vi "OE_Mis_time.vi"(7 "Seelected date":timestamp=timestamp(3772872308.6086583 s since 1904-01-01), 8 "error in (no error)":errorcluster, 10 "Cluster in":T1={"connection reference"=refnum, "Net Avai time (Min)"=0, "pLAN dATE datA"=[], "Data by plan date, shift, product"=[], "BreakDownd Data"=[], "Raw rejection Data"=[], "mislanius times shift 1"={"Lunch Time From"=timestamp(3772871904.6410136 s since 1904-01-01), "Lunch Time To"=timestamp(3772871909.6739416 s since 1904-01-01), "Tea Time From"=timestamp(3772871914.1118393 s since 1904-01-01), "Tea Time To"=timestamp(3772871912.0217314 s since 1904-01-01), "Clean Time From"=timestamp(3772871918.5572615 s since 1904-01-01), "Clean Time To"=timestamp(3772871916.1777034 s since 1904-01-01), "Meeting Time From"=timestamp(3772871920.7462983 s since 1904-01-01), "Meeting Time To"=timestamp(3772871922.664581 s since 1904-01-01), "Dev/Other Time From"=timestamp(3772871924.9359455 s since 1904-01-01), "Dev/Other Time To"=timestamp(3772871926.9172926 s since 1904-01-01), "Meeting"=TRUE, "Dev/Other"=TRUE}, "mislanius times shift 2"={"Lunch Time From"=timestamp(3772871937.417959 s since 1904-01-01), "Lunch Time To"=timestamp(3772871939.5655127 s since 1904-01-01), "Tea Time From"=timestamp(3772871941.53232 s since 1904-01-01), "Tea Time To"=timestamp(3772871944.2390895 s since 1904-01-01), "Clean Time From"=timestamp(3772871947.9368706 s since 1904-01-01), "Clean Time To"=timestamp(3772871950.09432 s since 1904-01-01), "Meeting Time From"=timestamp(3772871952.5211887 s since 1904-01-01), "Meeting Time To"=timestamp(3772871954.4985256 s since 1904-01-01), "Dev/Other Time From"=timestamp(3772871934.6783137 s since 1904-01-01), "Dev/Other Time To"=timestamp(3772871932.403295 s since 1904-01-01), "Meeting"=TRUE, "Dev/Other"=TRUE}} {"mislanius times shift 2"."Lunch Time From" format="%<%.X %x>T"; "mislanius times shift 2"."Lunch Time To" format="%<%.X %x>T"; "mislanius times shift 2"."Tea Time From" format="%<%.X %x>T"; "mislanius times shift 2"."Tea Time To" format="%<%.X %x>T"; "mislanius times shift 2"."Clean Time From" format="%<%.X %x>T"; "mislanius times shift 2"."Clean Time To" format="%<%.X %x>T"; "mislanius times shift 2"."Meeting Time From" format="%<%.X %x>T"; "mislanius times shift 2"."Meeting Time To" format="%<%.X %x>T"; "mislanius times shift 2"."Dev/Other Time From" format="%<%.X %x>T"; "mislanius times shift 2"."Dev/Other Time To" format="%<%.X %x>T"; "mislanius times shift 1"."Lunch Time From" format="%<%.X %x>T"; "mislanius times shift 1"."Lunch Time To" format="%<%.X %x>T"; "mislanius times shift 1"."Tea Time From" format="%<%.X %x>T"; "mislanius times shift 1"."Tea Time To" format="%<%.X %x>T"; "mislanius times shift 1"."Clean Time From" format="%<%.X %x>T"; "mislanius times shift 1"."Clean Time To" format="%<%.X %x>T"; "mislanius times shift 1"."Meeting Time From" format="%<%.X %x>T"; "mislanius times shift 1"."Meeting Time To" format="%<%.X %x>T"; "mislanius times shift 1"."Dev/Other Time From" format="%<%.X %x>T"; "mislanius times shift 1"."Dev/Other Time To" format="%<%.X %x>T"}, 11 "appended path":path) -> (0 "error out":errorcluster, 1 "Cluster out":T1={"connection reference"=refnum, "Net Avai time (Min)"=0, "pLAN dATE datA"=[], "Data by plan date, shift, product"=[], "BreakDownd Data"=[], "Raw rejection Data"=[], "mislanius times shift 1"={"Lunch Time From"=timestamp(0 s since 1904-01-01), "Lunch Time To"=timestamp(0 s since 1904-01-01), "Tea Time From"=timestamp(0 s since 1904-01-01), "Tea Time To"=timestamp(0 s since 1904-01-01), "Clean Time From"=timestamp(0 s since 1904-01-01), "Clean Time To"=timestamp(0 s since 1904-01-01), "Meeting Time From"=timestamp(0 s since 1904-01-01), "Meeting Time To"=timestamp(0 s since 1904-01-01), "Dev/Other Time From"=timestamp(0 s since 1904-01-01), "Dev/Other Time To"=timestamp(0 s since 1904-01-01), "Meeting"=FALSE, "Dev/Other"=TRUE}, "mislanius times shift 2"={"Lunch Time From"=timestamp(0 s since 1904-01-01), "Lunch Time To"=timestamp(0 s since 1904-01-01), "Tea Time From"=timestamp(0 s since 1904-01-01), "Tea Time To"=timestamp(0 s since 1904-01-01), "Clean Time From"=timestamp(0 s since 1904-01-01), "Clean Time To"=timestamp(0 s since 1904-01-01), "Meeting Time From"=timestamp(0 s since 1904-01-01), "Meeting Time To"=timestamp(0 s since 1904-01-01), "Dev/Other Time From"=timestamp(0 s since 1904-01-01), "Dev/Other Time To"=timestamp(0 s since 1904-01-01), "Meeting"=FALSE, "Dev/Other"=TRUE}} {"mislanius times shift 2"."Lunch Time From" format="%<%.X %x>T"; "mislanius times shift 2"."Lunch Time To" format="%<%.X %x>T"; "mislanius times shift 2"."Tea Time From" format="%<%.X %x>T"; "mislanius times shift 2"."Tea Time To" format="%<%.X %x>T"; "mislanius times shift 2"."Clean Time From" format="%<%.X %x>T"; "mislanius times shift 2"."Clean Time To" format="%<%.X %x>T"; "mislanius times shift 2"."Meeting Time From" format="%<%.X %x>T"; "mislanius times shift 2"."Meeting Time To" format="%<%.X %x>T"; "mislanius times shift 2"."Dev/Other Time From" format="%<%.X %x>T"; "mislanius times shift 2"."Dev/Other Time To" format="%<%.X %x>T"; "mislanius times shift 1"."Lunch Time From" format="%<%.X %x>T"; "mislanius times shift 1"."Lunch Time To" format="%<%.X %x>T"; "mislanius times shift 1"."Tea Time From" format="%<%.X %x>T"; "mislanius times shift 1"."Tea Time To" format="%<%.X %x>T"; "mislanius times shift 1"."Clean Time From" format="%<%.X %x>T"; "mislanius times shift 1"."Clean Time To" format="%<%.X %x>T"; "mislanius times shift 1"."Meeting Time From" format="%<%.X %x>T"; "mislanius times shift 1"."Meeting Time To" format="%<%.X %x>T"; "mislanius times shift 1"."Dev/Other Time From" format="%<%.X %x>T"; "mislanius times shift 1"."Dev/Other Time To" format="%<%.X %x>T"})   [LabVIEW 2017]
uses:
  Controls/OE_screen_cluster.ctl
  <vilib>/addons/database/Connection.llb/Conn ObjectReference.ctl
  <vilib>/addons/database/NI_Database_API.lvlib
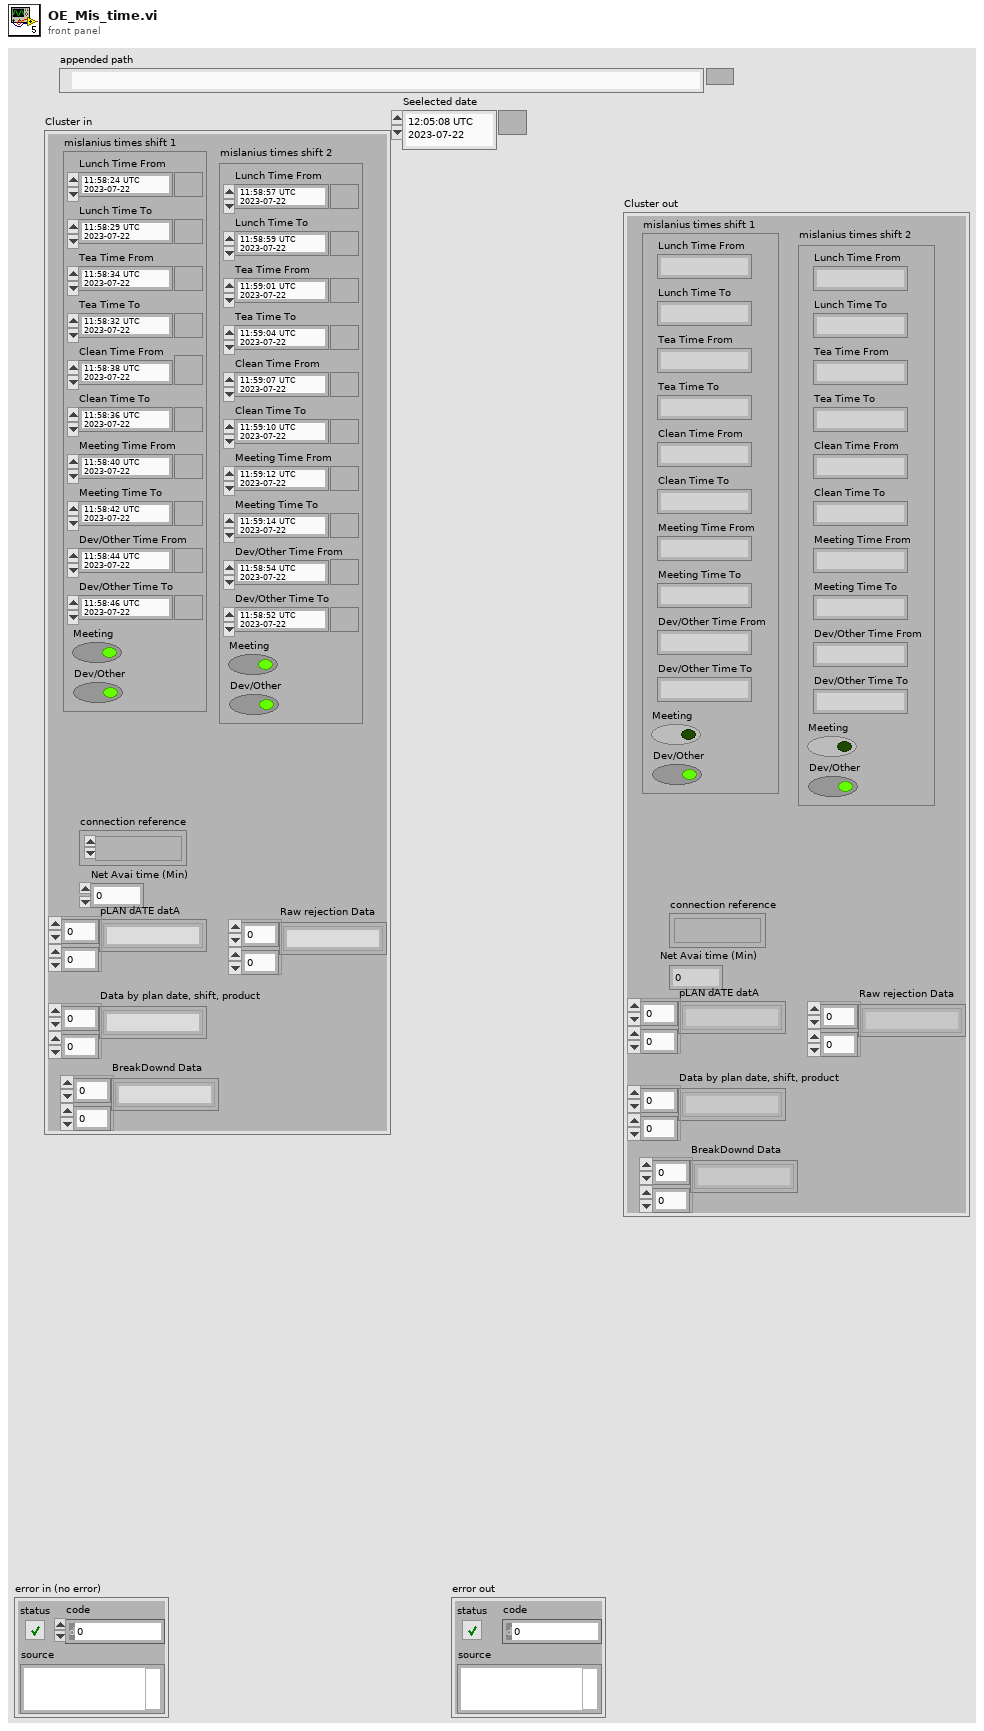
[diagram p1: front panel]
types:
  T1 = typedef "OE_screen_cluster.ctl" = cluster{"connection reference":T2, "Net Avai time (Min)":i32, "pLAN dATE datA":string[][], "Data by plan date, shift, product":string[][], "BreakDownd Data":string[][], "Raw rejection Data":string[][], "mislanius times shift 1":cluster{"Lunch Time From":timestamp, "Lunch Time To":timestamp, "Tea Time From":timestamp, "Tea Time To":timestamp, "Clean Time From":timestamp, "Clean Time To":timestamp, "Meeting Time From":timestamp, "Meeting Time To":timestamp, "Dev/Other Time From":timestamp, "Dev/Other Time To":timestamp, "Meeting":bool, "Dev/Other":bool}, "mislanius times shift 2":cluster{"Lunch Time From":timestamp, "Lunch Time To":timestamp, "Tea Time From":timestamp, "Tea Time To":timestamp, "Clean Time From":timestamp, "Clean Time To":timestamp, "Meeting Time From":timestamp, "Meeting Time To":timestamp, "Dev/Other Time From":timestamp, "Dev/Other Time To":timestamp, "Meeting":bool, "Dev/Other":bool}}
  T2 = typedef "NI_Database_API.lvlib/Conn ObjectReference.ctl" = refnum<k1>
  T3 = enum16{"open", "replace", "create", "open or create", "replace or create", "replace or create with confirmation"}
  T4 = cluster{"unsigned 64bit integer":u64, "unsigned 64bit integer 2":u64, "unsigned 64bit integer 3":u64, "unsigned 64bit integer 4":u64, "unsigned 64bit integer 5":u64, "unsigned 64bit integer 6":u64, "unsigned 64bit integer 7":u64, "unsigned 64bit integer 8":u64, "unsigned 64bit integer 9":u64, "unsigned 64bit integer 10":u64, "Meeting":bool, "Dev/other 1":bool, "unsigned 64bit integer 11":u64, "unsigned 64bit integer 12":u64, "unsigned 64bit integer 13":u64, "unsigned 64bit integer 14":u64, "unsigned 64bit integer 15":u64, "unsigned 64bit integer 16":u64, "unsigned 64bit integer 17":u64, "unsigned 64bit integer 18":u64, "unsigned 64bit integer 19":u64, "unsigned 64bit integer 20":u64, "Meeting 2":bool, "Dev/other 2":bool}
  T5 = cluster{"Lunch Time From":timestamp, "Lunch Time To":timestamp, "Tea Time From":timestamp, "Tea Time To":timestamp, "Clean Time From":timestamp, "Clean Time To":timestamp, "Meeting Time From":timestamp, "Meeting Time To":timestamp, "Dev/Other Time From":timestamp, "Dev/Other Time To":timestamp, "Meeting":bool, "Dev/Other":bool}
  T6 = typedef "LVDateTimeRec.ctl" = cluster{"fractional second":dbl, "second":i32, "minute":i32, "hour":i32, "day of month":i32, "month":i32, "year":i32, "day of week":i32, "day of year":i32, "DST":i32}
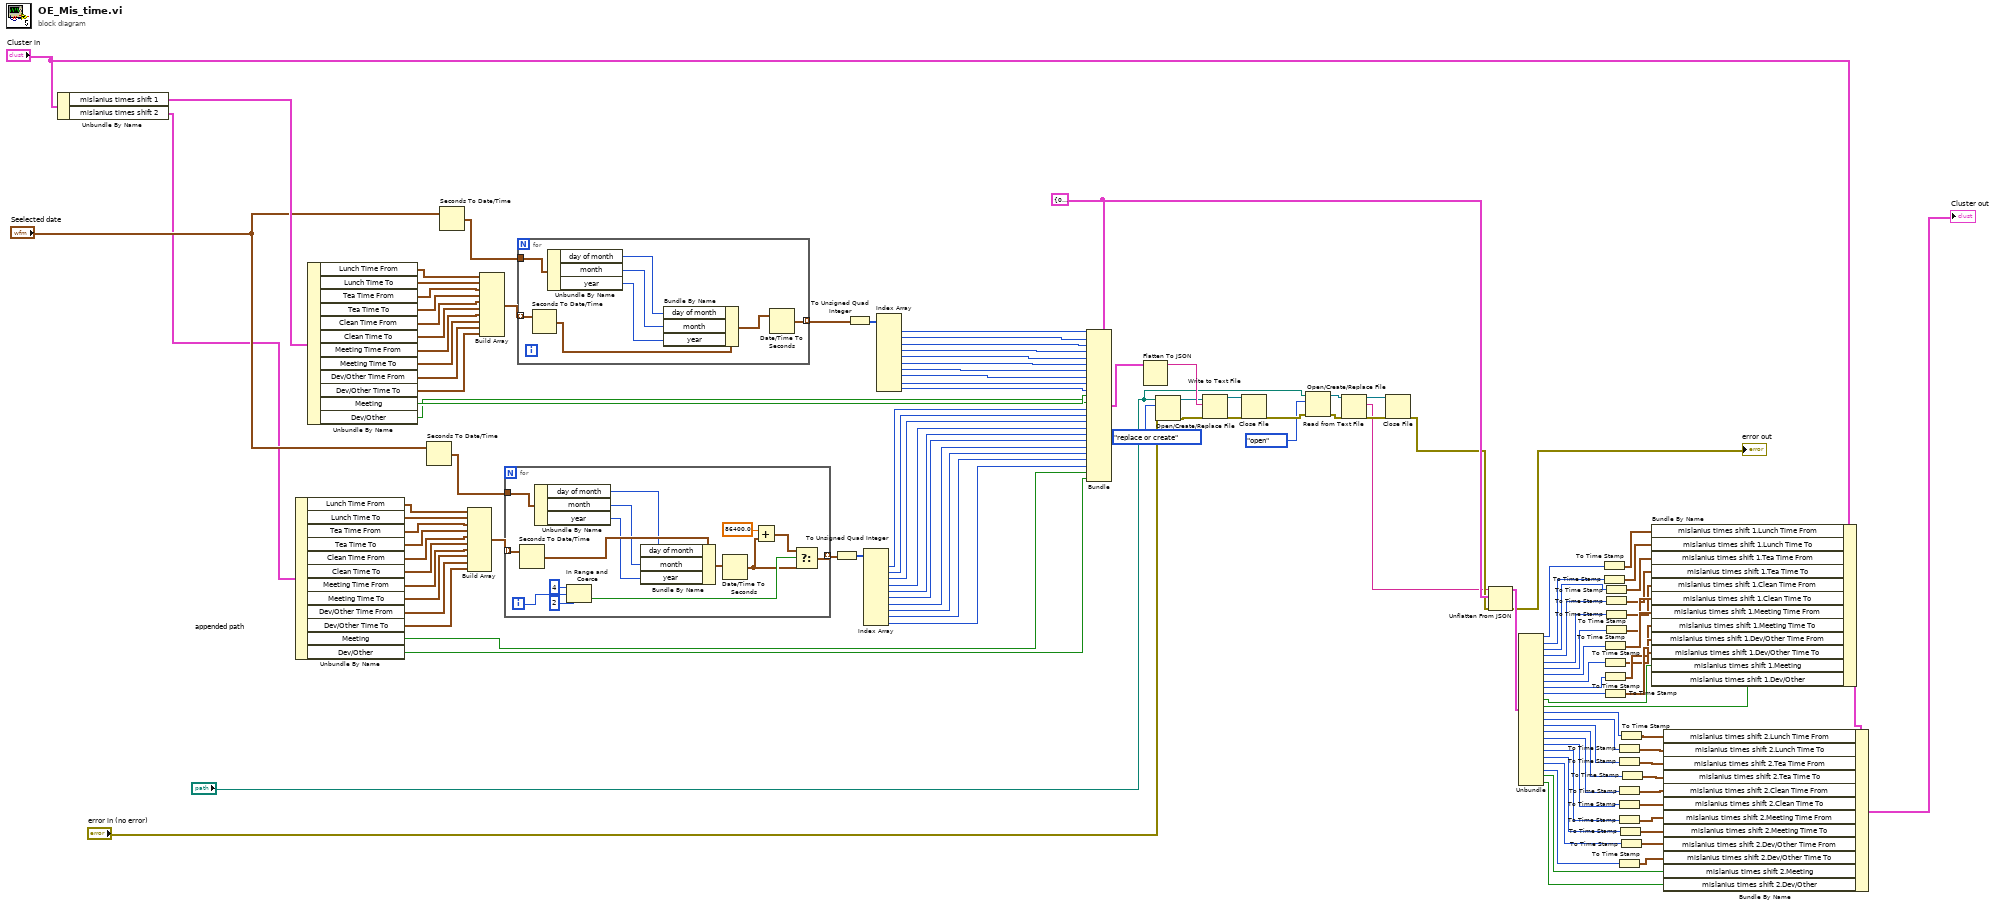
[diagram p0: block diagram]
diagram:
  w93 = T4 {"unsigned 64bit integer"=0, "unsigned 64bit integer 2"=0, "unsigned 64bit integer 3"=0, "unsigned 64bit integer 4"=0, "unsigned 64bit integer 5"=0, "unsigned 64bit integer 6"=0, "unsigned 64bit integer 7"=0, "unsigned 64bit integer 8"=0, "unsigned 64bit integer 9"=0, "unsigned 64bit integer 10"=0, "Meeting"=FALSE, "Dev/other 1"=FALSE, "unsigned 64bit integer 11"=0, "unsigned 64bit integer 12"=0, "unsigned 64bit integer 13"=0, "unsigned 64bit integer 14"=0, "unsigned 64bit integer 15"=0, "unsigned 64bit integer 16"=0, "unsigned 64bit integer 17"=0, "unsigned 64bit integer 18"=0, "unsigned 64bit integer 19"=0, "unsigned 64bit integer 20"=0, "Meeting 2"=FALSE, "Dev/other 2"=FALSE} ("input cluster")
  n1 = Unbundle By Name("Cluster in") -> ("mislanius times shift 1"=w81:T5, "mislanius times shift 2"=w41:T5)
  n2 = Unbundle By Name(w41) -> ("Lunch Time From"=w43:timestamp, "Lunch Time To"=w45:timestamp, "Tea Time From"=w46:timestamp, "Tea Time To"=w47:timestamp, "Clean Time From"=w48:timestamp, "Clean Time To"=w49:timestamp, "Meeting Time From"=w50:timestamp, "Meeting Time To"=w51:timestamp, "Dev/Other Time From"=w52:timestamp, "Dev/Other Time To"=w53:timestamp, "Meeting"=w38:bool, "Dev/Other"=w37:bool)
  n3 = Unbundle By Name(w81) -> ("Lunch Time From"=w80:timestamp, "Lunch Time To"=w78:timestamp, "Tea Time From"=w77:timestamp, "Tea Time To"=w76:timestamp, "Clean Time From"=w75:timestamp, "Clean Time To"=w74:timestamp, "Meeting Time From"=w73:timestamp, "Meeting Time To"=w72:timestamp, "Dev/Other Time From"=w71:timestamp, "Dev/Other Time To"=w70:timestamp, "Meeting"=w40:bool, "Dev/Other"=w39:bool)
  n4 = Seconds To Date/Time(time stamp (now)="Seelected date") -> (date time rec=w54:T6)  [unwired: 1 in]
  n5 = Seconds To Date/Time(time stamp (now)="Seelected date") -> (date time rec=w69:T6)  [unwired: 1 in]
  n6 = Build Array(w43, w45, w46, w47, w48, w49, w50, w51, w52, w53) -> (w44:timestamp[])
  n7 = Build Array(w80, w78, w77, w76, w75, w74, w73, w72, w71, w70) -> (w79:timestamp[])
  n8 = for {
    tunnel: w44 -> [w135] mode=indexing
    tunnel: w54 -> [w127]
    tunnel: [w124] -> w55 mode=indexing
    i -> [w130]
    n9 = Seconds To Date/Time(time stamp (now)=w135) -> (date time rec=w137:T6)  [unwired: 1 in]
    n10 = Unbundle By Name(w127) -> ("day of month"=w129:i32, "month"=w134:i32, "year"=w133:i32)
    n11 = In Range and Coerce(upper limit=4, x=w130, lower limit=2) -> (In Range?=w126:bool)  [unwired: 1 out]
    n12 = Bundle By Name(cluster=w137, "day of month"=w129, "month"=w134, "year"=w133) -> (w136:T6)
    n13 = Date/Time To Seconds(2:w136) -> (0:w123:timestamp)  [unwired: 1 in]
    n14 = Add(x=86400.0 ("x-y 2"), y=w123) -> (x+y=w125:timestamp)
    n15 = Select(t=w125, s=w126, f=w123) -> (s? t:f=w124:timestamp)
  }
  n16 = for {
    tunnel: w79 -> [w143] mode=indexing
    tunnel: w69 -> [w142]
    tunnel: [w138] -> w68 mode=indexing
    n17 = Seconds To Date/Time(time stamp (now)=w143) -> (date time rec=w145:T6)  [unwired: 1 in]
    n18 = Unbundle By Name(w142) -> ("day of month"=w141:i32, "month"=w140:i32, "year"=w139:i32)
    n19 = Bundle By Name(cluster=w145, "day of month"=w141, "month"=w140, "year"=w139) -> (w144:T6)
    n20 = Date/Time To Seconds(2:w144) -> (0:w138:timestamp)  [unwired: 1 in]
  }
  n21 = To Unsigned Quad Integer(1:w55) -> (0:w56:u64[])
  n22 = To Unsigned Quad Integer(1:w68) -> (0:w67:u64[])
  n23 = Index Array(array=w56) -> (element #1=w27:u64, element #2=w28:u64, element #3=w29:u64, element #4=w30:u64, element #5=w31:u64, element #6=w32:u64, element #7=w33:u64, element #8=w34:u64, element #9=w35:u64, element #10=w36:u64)  [unwired: 10 in]
  n24 = Index Array(array=w67) -> (element #1=w66:u64, element #2=w65:u64, element #3=w64:u64, element #4=w63:u64, element #5=w62:u64, element #6=w61:u64, element #7=w60:u64, element #8=w59:u64, element #9=w58:u64, element #10=w57:u64)  [unwired: 10 in]
  n25 = Bundle(cluster=w93, "unsigned 64bit integer"=w66, "unsigned 64bit integer 2"=w65, "unsigned 64bit integer 3"=w64, "unsigned 64bit integer 4"=w63, "unsigned 64bit integer 5"=w62, "unsigned 64bit integer 6"=w61, "unsigned 64bit integer 7"=w60, "unsigned 64bit integer 8"=w59, "unsigned 64bit integer 9"=w58, "unsigned 64bit integer 10"=w57, "Meeting"=w40, "Dev/other 1"=w39, "unsigned 64bit integer 11"=w27, "unsigned 64bit integer 12"=w28, "unsigned 64bit integer 13"=w29, "unsigned 64bit integer 14"=w30, "unsigned 64bit integer 15"=w31, "unsigned 64bit integer 16"=w32, "unsigned 64bit integer 17"=w33, "unsigned 64bit integer 18"=w34, "unsigned 64bit integer 19"=w35, "unsigned 64bit integer 20"=w36, "Meeting 2"=w38, "Dev/other 2"=w37) -> (w118:T4)
  n26 = Flatten To JSON(anything=w118) -> (JSON string=w92:string)  [unwired: 2 in, 1 out]
  n27 = Open/Create/Replace File(file path (use dialog)="appended path", error in="error in (no error)", operation (0:open)=T3."replace or create") -> (refnum out=w88:refnum<file>, error out=w121:errorcluster)  [unwired: 3 in, 1 out]
  n28 = Write to Text File(file (use dialog)=w88, text=w92, error in=w121) -> (refnum out=w86:refnum<file>, error out=w87:errorcluster)  [unwired: 1 in, 1 out]
  n29 = Close File(refnum=w86, error in=w87) -> (error out=w85:errorcluster)  [unwired: 1 out]
  n30 = Open/Create/Replace File(file path (use dialog)="appended path", error in=w85, operation (0:open)=T3."open") -> (refnum out=w83:refnum<file>, error out=w84:errorcluster)  [unwired: 3 in, 1 out]
  n31 = Read from Text File(file (use dialog)=w83, error in=w84) -> (refnum out=w120:refnum<file>, text=w89:string, error out=w119:errorcluster)  [unwired: 2 in, 1 out]
  n32 = Close File(refnum=w120, error in=w119) -> (error out=w91:errorcluster)  [unwired: 1 out]
  n33 = Unflatten From JSON(JSON string=w89, type and defaults=w93, error in (no error)=w91) -> (value=w107:T4, error out=→"error out":errorcluster)  [unwired: 4 in]
  n34 = Unbundle(w107) -> ("unsigned 64bit integer"=w24:u64, "unsigned 64bit integer 2"=w23:u64, "unsigned 64bit integer 3"=w22:u64, "unsigned 64bit integer 4"=w21:u64, "unsigned 64bit integer 5"=w20:u64, "unsigned 64bit integer 6"=w19:u64, "unsigned 64bit integer 7"=w18:u64, "unsigned 64bit integer 8"=w17:u64, "unsigned 64bit integer 9"=w16:u64, "unsigned 64bit integer 10"=w15:u64, "Meeting"=w26:bool, "Dev/other 1"=w25:bool, "unsigned 64bit integer 11"=w4:u64, "unsigned 64bit integer 12"=w5:u64, "unsigned 64bit integer 13"=w6:u64, "unsigned 64bit integer 14"=w7:u64, "unsigned 64bit integer 15"=w8:u64, "unsigned 64bit integer 16"=w9:u64, "unsigned 64bit integer 17"=w10:u64, "unsigned 64bit integer 18"=w11:u64, "unsigned 64bit integer 19"=w12:u64, "unsigned 64bit integer 20"=w13:u64, "Meeting 2"=w14:bool, "Dev/other 2"=w82:bool)
  n35 = To Time Stamp(1:w24) -> (0:w108:timestamp)
  n36 = To Time Stamp(1:w23) -> (0:w109:timestamp)
  n37 = To Time Stamp(1:w18) -> (0:w114:timestamp)
  n38 = To Time Stamp(1:w17) -> (0:w115:timestamp)
  n39 = To Time Stamp(1:w16) -> (0:w116:timestamp)
  n40 = To Time Stamp(1:w15) -> (0:w117:timestamp)
  n41 = To Time Stamp(1:w22) -> (0:w110:timestamp)
  n42 = To Time Stamp(1:w21) -> (0:w111:timestamp)
  n43 = To Time Stamp(1:w20) -> (0:w112:timestamp)
  n44 = To Time Stamp(1:w19) -> (0:w113:timestamp)
  n45 = To Time Stamp(1:w5) -> (0:w105:timestamp)
  n46 = To Time Stamp(1:w6) -> (0:w104:timestamp)
  n47 = To Time Stamp(1:w9) -> (0:w101:timestamp)
  n48 = To Time Stamp(1:w10) -> (0:w100:timestamp)
  n49 = To Time Stamp(1:w8) -> (0:w102:timestamp)
  n50 = To Time Stamp(1:w13) -> (0:w97:timestamp)
  n51 = To Time Stamp(1:w11) -> (0:w99:timestamp)
  n52 = To Time Stamp(1:w4) -> (0:w106:timestamp)
  n53 = To Time Stamp(1:w12) -> (0:w98:timestamp)
  n54 = To Time Stamp(1:w7) -> (0:w103:timestamp)
  n55 = Bundle By Name(cluster="Cluster in", "mislanius times shift 1.Lunch Time From"=w108, "mislanius times shift 1.Lunch Time To"=w109, "mislanius times shift 1.Tea Time From"=w110, "mislanius times shift 1.Tea Time To"=w111, "mislanius times shift 1.Clean Time From"=w112, "mislanius times shift 1.Clean Time To"=w113, "mislanius times shift 1.Meeting Time From"=w114, "mislanius times shift 1.Meeting Time To"=w115, "mislanius times shift 1.Dev/Other Time From"=w116, "mislanius times shift 1.Dev/Other Time To"=w117, "mislanius times shift 1.Meeting"=w26, "mislanius times shift 1.Dev/Other"=w25) -> (w96:T1)
  n56 = Bundle By Name(cluster=w96, "mislanius times shift 2.Lunch Time From"=w106, "mislanius times shift 2.Lunch Time To"=w105, "mislanius times shift 2.Tea Time From"=w104, "mislanius times shift 2.Tea Time To"=w103, "mislanius times shift 2.Clean Time From"=w102, "mislanius times shift 2.Clean Time To"=w101, "mislanius times shift 2.Meeting Time From"=w100, "mislanius times shift 2.Meeting Time To"=w99, "mislanius times shift 2.Dev/Other Time From"=w98, "mislanius times shift 2.Dev/Other Time To"=w97, "mislanius times shift 2.Meeting"=w14, "mislanius times shift 2.Dev/Other"=w82) -> (→"Cluster out":T1)
